vi "StatePowerManagement.vi"(0 "Master State In":T1(ring)) -> ()   [LabVIEW 2020]
doc: "This VI decides whether or not power should be diverted away from non-critical subsystems in an emergency or during certain periods of the match."
uses:
  GlobalDriverStationData.vi
  GlobalDrivebase.vi
  GlobalMiscellaneous.vi
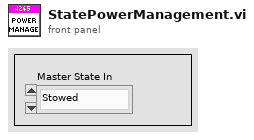
[diagram p1: front panel]
types:
  T1 = enum16{"Stowed", "Balancing", "Scoring", "Hoppering", "Ground", "Shelf"}
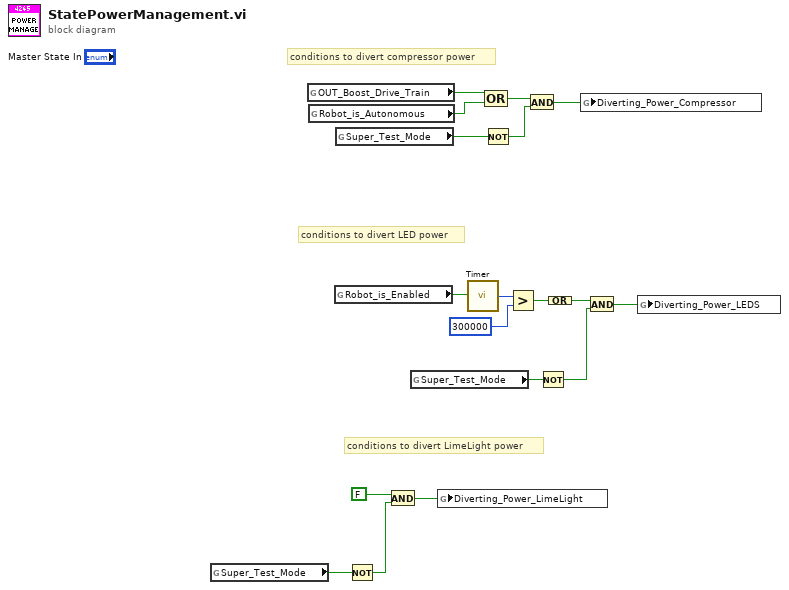
[diagram p0: block diagram]
diagram:
  # "conditions to divert LimeLight power"
  # "conditions to divert LED power"
  # "conditions to divert compressor power"
  n1 = global read "GlobalDriverStationData.vi" "Super_Test_Mode"() -> (w4:bool)
  n2 = global read "GlobalDrivebase.vi" "OUT_Boost_Drive_Train"() -> (w15:bool)
  n3 = global read "GlobalDriverStationData.vi" "Robot_is_Autonomous"() -> (w14:bool)
  n4 = global read "GlobalDriverStationData.vi" "Robot_is_Enabled"() -> (w12:bool)
  n5 = global read "GlobalDriverStationData.vi" "Super_Test_Mode"() -> (w6:bool)
  n6 = Not(x=w4) -> (.not. x?=w2:bool)
  n7 = And(x=FALSE, y=w2) -> (x .and. y?=w3:bool)
  n8 = global read "GlobalDriverStationData.vi" "Super_Test_Mode"() -> (w9:bool)
  n9 = global write "GlobalMiscellaneous.vi" "Diverting_Power_LimeLight"(w3) -> ()
  n10 = call "Timer.vi"("Reset Timer"=w12) -> ("Time (ms)"=w18:u32)
  n11 = Not(x=w6) -> (.not. x?=w5:bool)
  n12 = Compound Arithmetic op=OR(w15, w14) -> (w13:bool)
  n13 = Greater?(x=w18, y=u32 300000 ("x")) -> (0:w16:bool)
  n14 = And(x=w13, y=w5) -> (x .and. y?=w7:bool)
  n15 = Not(x=w9) -> (.not. x?=w8:bool)
  n16 = Compound Arithmetic op=OR(w16) -> (w11:bool)
  n17 = global write "GlobalMiscellaneous.vi" "Diverting_Power_Compressor"(w7) -> ()
  n18 = And(x=w11, y=w8) -> (x .and. y?=w10:bool)
  n19 = global write "GlobalMiscellaneous.vi" "Diverting_Power_LEDS"(w10) -> ()
